vi "p11y3MRWORLDWIDE.vi"(8 "error in (no error)":errorcluster, 10 "Tegevus":enum16{"lahuta", "liida", "alg", "loe"}(ring), 11 "algv22rtus":dbl) -> (0 "error out":errorcluster, 3 "v22rtus":dbl)   [LabVIEW 2020]
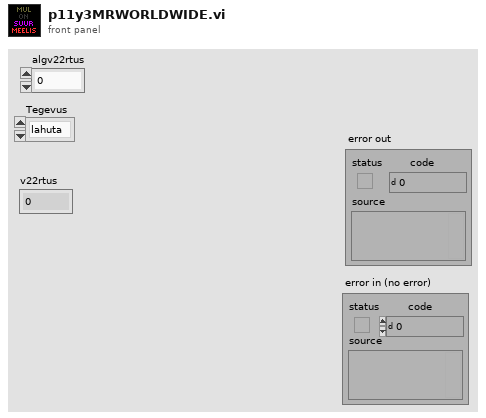
[diagram p1: front panel]
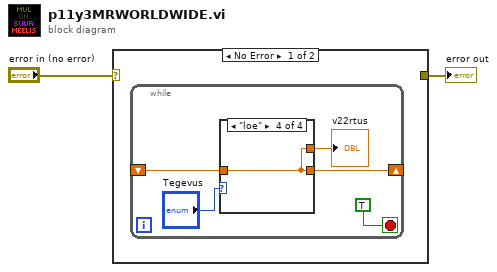
[diagram p0: block diagram]
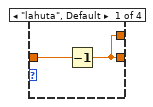
[diagram p2: hidden frame]
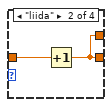
[diagram p3: hidden frame]
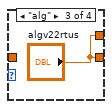
[diagram p4: hidden frame]
diagram:
  n1 = case shown="No Error" "error in (no error)" {
    selector: "error in (no error)" -> [_ w14]
    tunnel: [_ w14] -> w1
    frame No Error {
      n2 = while {
        shift-right: [w4] -> _
        shift-left: _ -> [w3]
        stop <- TRUE stop-if-true
        n3 = case shown="\"loe\"" "Tegevus" {
          tunnel: [w8 w10 "algv22rtus" w13] -> w5
          tunnel: [w8 w10 "algv22rtus" w13] -> w4
          tunnel: w3 -> [w9 w11 _ w13]
          frame "lahuta", Default {
            n4 = Decrement(x=w9) -> (x-1=w8:dbl)
          }
          frame "liida" {
            n5 = Increment(x=w11) -> (x+1=w10:dbl)
          }
          frame "alg" {
          }
          frame "loe" {
          }
        }
        "v22rtus" <- w5
      }
    }
    frame Error {
    }
  }
  "error out" <- w1
